vi "Data processor.vi"() -> ()   [LabVIEW 2016]
uses:
  <userlib>/LevyLab/LV to ITX/LVtoITX.lvclass
panel:
  out "N":cluster{"N1":dbl, "N2":dbl, "N3":dbl, "N4":dbl}={"N1"=0.0624995231628418, "N2"=0.0624995231628418, "N3"=0.0624995231628418, "N4"=0.0624995231628418} {"N4" format="%#_6p"; "N3" format="%#_6p"; "N2" format="%#_6p"; "N1" format="%#_6p"}
  out "E":dbl[][](graph)
  out "C vs D":cluster{dbl[], dbl[]}[](graph)
  out "A vs B":cluster{dbl[], dbl[]}[](graph)
  in  "index":T1={"A"=1, "B"=0, "C"=2, "D"=0, "E"=3, "N1"=0, "N2"=0, "N3"=0, "N4"=0}
  in  "length":i32=1
  in  "offset":i32
  in  "File or Folder Path":path=path "C:/"
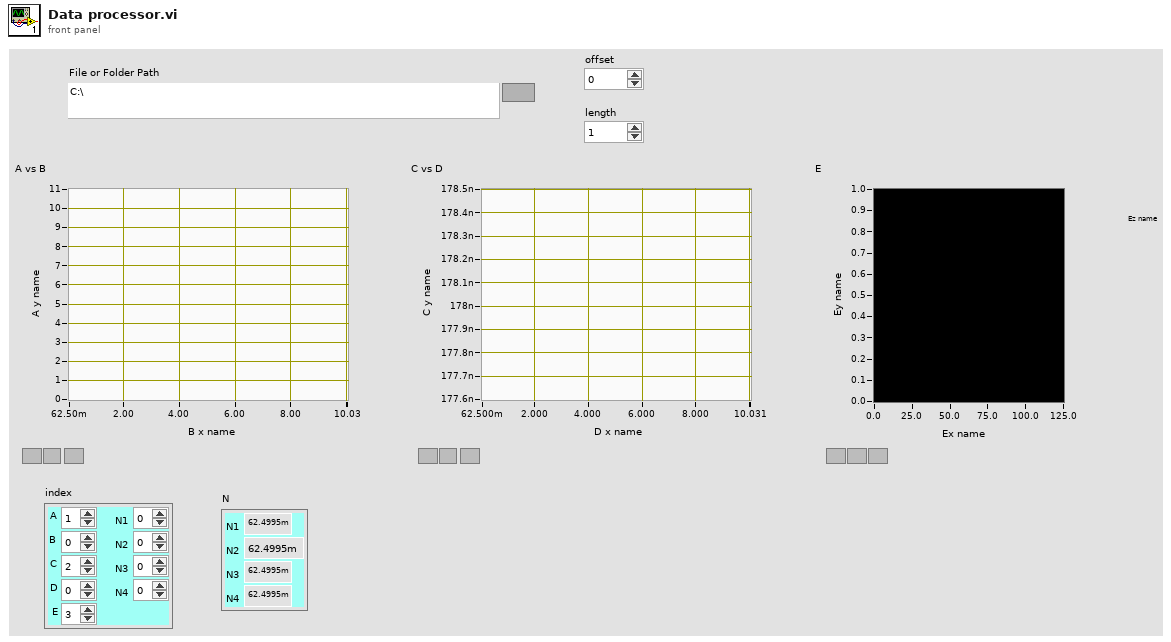
[diagram p1: front panel]
types:
  T1 = cluster{"A":i32, "B":i32, "C":i32, "D":i32, "E":i32, "N1":i32, "N2":i32, "N3":i32, "N4":i32}
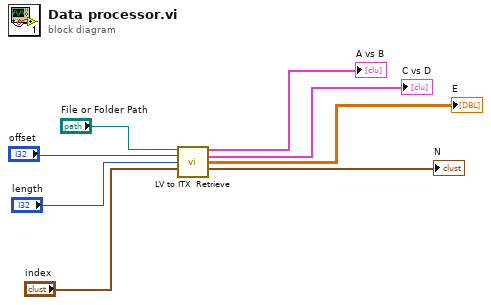
[diagram p0: block diagram]
diagram:
  n1 = call <userlib>:"LV to ITX  Retrieve.vi"("File or Folder Path"="File or Folder Path", "offset"="offset", "length"="length", "index"="index") -> ("A vs B"=→"A vs B":cluster{dbl[], dbl[]}[], "C vs D"=→"C vs D":cluster{dbl[], dbl[]}[], "E"=→"E":dbl[][], "N"=→"N":cluster{"N1":dbl, "N2":dbl, "N3":dbl, "N4":dbl})  [unwired: 7 in, 1 out]
